vi "ParseSteps.vi"(10 "StepIndicationString (//)":string="//", 11 "AscriptLines":string[](array[string])) -> (3 "Steps":T1(array[cluster]))   [LabVIEW 2015]
panel:
  out "AscriptName":string
  out "MetaData":string[](array[string])
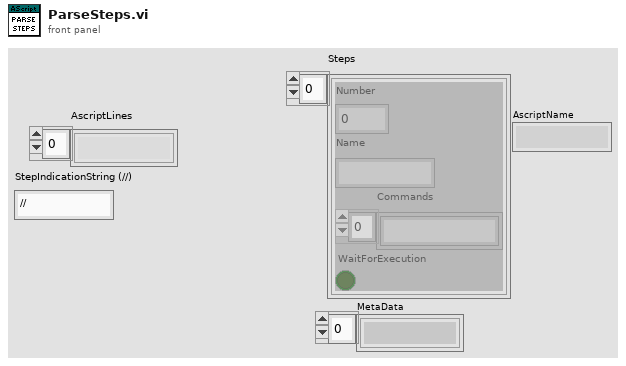
[diagram p1: front panel]
types:
  T1 = cluster{"Number":i32, "Name":string, "Commands":string[], "WaitForExecution":bool}[]
  T2 = cluster{"Number":i32, "Name":string, "Commands":string[], "WaitForExecution":bool}
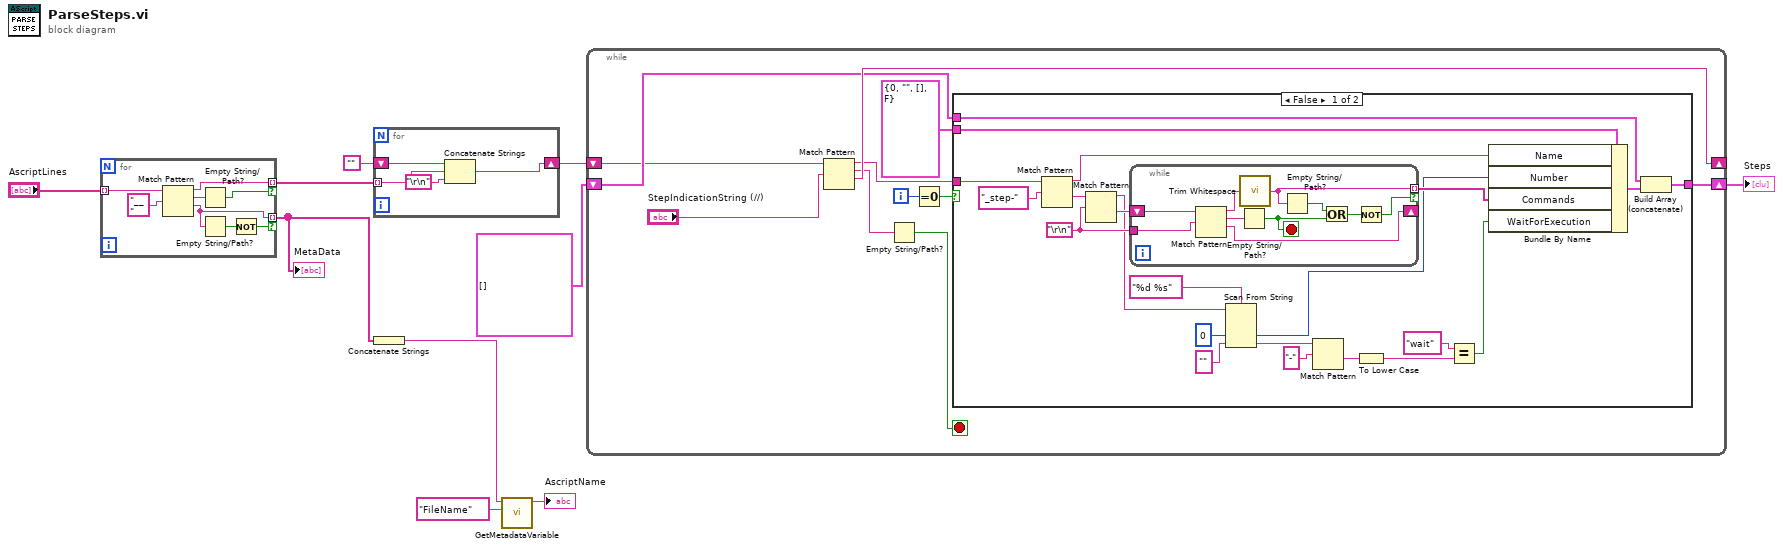
[diagram p0: block diagram]
diagram:
  n1 = for {
    tunnel: "AscriptLines" -> [w18] mode=indexing
    tunnel: [w16] -> w5 mode=indexing if=w11
    tunnel: [w12] -> w4 mode=indexing if=w13
    n2 = Match Pattern(string=w18, regular expression="__") -> (before substring=w16:string, match substring=w15:string, after substring=w12:string)  [unwired: 1 in, 1 out]
    n3 = Empty String/Path?(string/path=w15) -> (empty?=w11:bool)
    n4 = Empty String/Path?(string/path=w12) -> (empty?=w14:bool)
    n5 = Not(x=w14) -> (.not. x?=w13:bool)
  }
  "MetaData" <- w4
  n6 = for {
    tunnel: w5 -> [w21] mode=indexing
    shift-right: [w20] -> w10
    shift-left: "" -> [w22]
    n7 = Concatenate Strings(w22, w21, "\r\n") -> (w20:string)
  }
  n8 = Concatenate Strings(w4) -> (w3:string)
  n9 = call "GetMetadataVariable.vi"("Variable name"="FileName", "input string"=w3) -> ("Variable Value"=→"AscriptName":string)  [unwired: 7 in, 2 out]
  n10 = while {
    shift-right: [w27] -> w8
    shift-left: T1 [] -> [w29]
    shift-right: [w32] -> _
    shift-left: w10 -> [w23]
    i -> [w31]
    stop <- w25 stop-if-true
    n11 = Match Pattern(string=w23, regular expression="StepIndicationString (//)") -> (before substring=w30:string, match substring=w26:string, after substring=w32:string)  [unwired: 1 in, 1 out]
    n12 = Empty String/Path?(string/path=w26) -> (empty?=w25:bool)
    n13 = Equal To 0?(x=w31) -> (x = 0?=w24:bool)
    n14 = case shown="False" w24 {
      tunnel: w30 -> [w55 _]
      tunnel: w29 -> [w47 w66]
      tunnel: T2 {"Number"=0, "Name"="", "Commands"=[], "WaitForExecution"=FALSE} ("Step") -> [w53 _]
      tunnel: [w46 w66] -> w27
      frame False {
        w45 = "\r\n"
        n15 = Match Pattern(string=w55, regular expression="_step-") -> (before substring=w52:string, after substring=w51:string)  [unwired: 1 in, 2 out]
        n16 = Match Pattern(string=w51, regular expression=w45) -> (before substring=w44:string, after substring=w50:string)  [unwired: 1 in, 2 out]
        n17 = while {
          shift-right: [w63] -> _
          shift-left: w50 -> [w65]
          tunnel: w45 -> [w64]
          tunnel: [w56] -> w49 mode=indexing if=w61
          stop <- w58 stop-if-true
          n18 = Match Pattern(string=w65, regular expression=w64) -> (before substring=w57:string, match substring=w62:string, after substring=w63:string)  [unwired: 1 in, 1 out]
          n19 = Empty String/Path?(string/path=w62) -> (empty?=w58:bool)
          n20 = call <vilib>:"Trim Whitespace.vi"("string"=w57) -> ("trimmed string"=w56:string)  [unwired: 1 in]
          n21 = Empty String/Path?(string/path=w56) -> (empty?=w59:bool)
          n22 = Or(x=w59, y=w58) -> (x .or. y?=w60:bool)
          n23 = Not(x=w60) -> (.not. x?=w61:bool)
        }
        n24 = Scan From String(format string="%d %s", input string=w44, default 1=0 ("default value 1"), default 2="" ("default value 2")) -> (output 1=w42:i32, output 2=w41:string)  [unwired: 2 in, 3 out]
        n25 = Match Pattern(string=w41, regular expression="-") -> (after substring=w39:string)  [unwired: 1 in, 3 out]
        n26 = To Lower Case(string=w39) -> (all lower case string=w38:string)
        n27 = Equal?(x="wait", y=w38) -> (x = y?=w36:bool)
        n28 = Bundle By Name(cluster=w53, "Name"=w52, "Number"=w42, "Commands"=w49, "WaitForExecution"=w36) -> (w48:T2)
        n29 = Build Array (concatenate)(w47, w48) -> (w46:T1)
      }
      frame True {
      }
    }
  }
  "Steps" <- w8
